vi "Experiment Driver.vi"(0 "Experiment VI Reference":refnum<vi>) -> ()   [LabVIEW 2013]
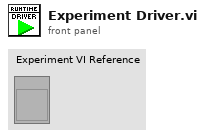
[diagram p1: front panel]
types:
  T1 = typedef "Semaphore RefNum" = refnum<k1>
  T2 = typedef "Runtime Queue.ctl" = refnum<queue>
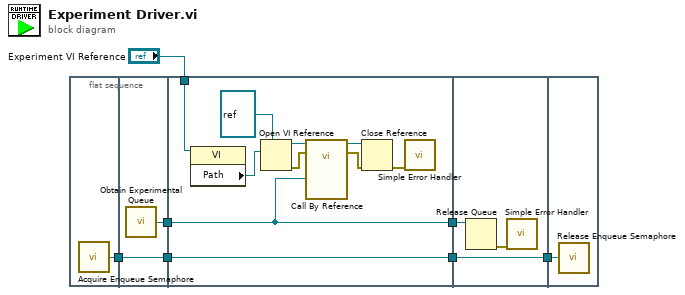
[diagram p0: block diagram]
diagram:
  n1 = flat-sequence {
    tunnel: [w8] -> w7
    tunnel: w7 -> [w10]
    tunnel: [w10] -> w6
    tunnel: [w9] -> w5
    tunnel: w6 -> [w20]
    tunnel: w5 -> [w11]
    tunnel: [w20] -> w4
    tunnel: [w11] -> w3
    tunnel: "Experiment VI Reference" -> [w12]
    tunnel: [w23] -> w2
    tunnel: w4 -> [w23]
    tunnel: w3 -> [w22]
    tunnel: w2 -> [w24]
    frame #0 {
      n2 = call "Acquire Enqueue Semaphore.vi"() -> ("Semaphore Reference"=w8:T1)
    }
    frame #1 {
      n3 = call "Obtain Experimental Queue.vi"() -> ("Experimental Queue"=w9:T2)
    }
    frame #2 {
      n4 = property class="VI"(reference=w12) -> ("Path"=w18:path)  [unwired: 1 in, 2 out]
      n5 = Open VI Reference(type specifier VI Refnum (for type only)=refnum<vi> refnum, vi path=w18) -> (vi reference=w17:refnum<vi>, error out=w16:errorcluster)  [unwired: 4 in]
      n6 = call-by-ref "?"(reference=w17, error in=w16, "Experimental Queue"=w11) -> (reference out=w15:refnum<vi>, error out=w14:errorcluster)
      n7 = Close Reference(reference=w15, error in (no error)=w14) -> (error out=w13:errorcluster)
      n8 = call <vilib>:"Simple Error Handler.vi"("error in (no error)"=w13) -> ()  [unwired: 4 in, 5 out]
    }
    frame #3 {
      n9 = Release Queue(queue=w22) -> (error out=w21:errorcluster)  [unwired: 2 in, 2 out]
      n10 = call <vilib>:"Simple Error Handler.vi"("error in (no error)"=w21) -> ()  [unwired: 4 in, 5 out]
    }
    frame #4 {
      n11 = call "Release Enqueue Semaphore.vi"("Semaphore Reference"=w24) -> ()
    }
  }
